vi "事件结构的使用(上).vi"() -> ()   [LabVIEW 2018]
panel:
  out "x-y":dbl
  in  "旋钮":dbl(knob) scale=0.0..10.0
  out "闪烁":bool
  out "布尔 2":bool
  out "滑动杆":dbl(slide) scale=0.0..10.0
  in  "布尔":bool
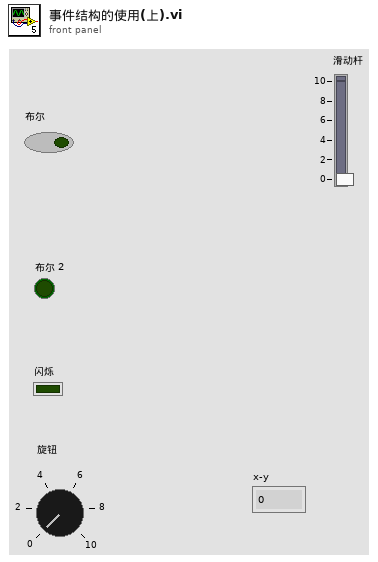
[diagram p1: front panel]
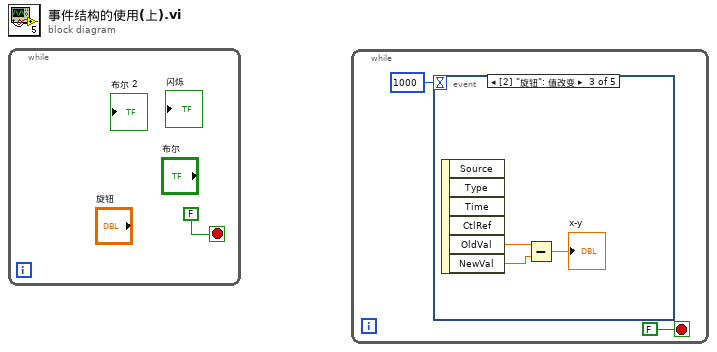
[diagram p0: block diagram]
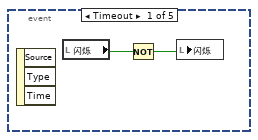
[diagram p2: hidden frame]
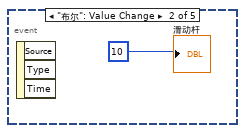
[diagram p3: hidden frame]
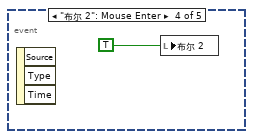
[diagram p4: hidden frame]
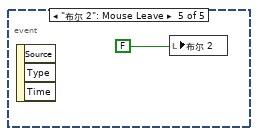
[diagram p5: hidden frame]
diagram:
  n1 = while {
    stop <- FALSE stop-if-true
  }
  n2 = while {
    stop <- FALSE stop-if-true
    n3 = event shown="[2] \"旋钮\": 值改变" {
      selector: _ -> [_ _ _ _ _]
      dyn-events: _ -> [_ _ _ _ _]
      timeout: 1000 -> [_ _ _ _ _]
      event Timeout {
        n4 = event-data() -> ()  [unwired: 1 in, 3 out]
        n5 = local read "闪烁"() -> (w5:bool)
        n6 = Not(x=w5) -> (.not. x?=w4:bool)
        n7 = local write "闪烁"(w4) -> ()
      }
      event "布尔": Value Change {
        n8 = event-data() -> ()  [unwired: 1 in, 3 out]
        "滑动杆" <- 10
      }
      event "旋钮": Value Change {
        n9 = event-data() -> ("OldVal"=w9:dbl, "NewVal"=w8:dbl)  [unwired: 1 in, 4 out]
        n10 = Subtract(x=w9, y=w8) -> (x-y=→"x-y":dbl)
      }
      event "布尔 2": Mouse Enter {
        n11 = event-data() -> ()  [unwired: 1 in, 3 out]
        n12 = local write "布尔 2"(TRUE) -> ()
      }
      event "布尔 2": Mouse Leave {
        n13 = event-data() -> ()  [unwired: 1 in, 3 out]
        n14 = local write "布尔 2"(FALSE) -> ()
      }
    }
  }
